vi "Add Abstract Message Attribute.vi"(8 "error in (no error)":errorcluster, 10 "Abstract Message Path":path, 11 "Target Actor in":refnum<vi>) -> (0 "error out":errorcluster, 2 "Abstract Message Control":refnum<vi>)   [LabVIEW 2020, in "Message Maker.lvlib"]
uses:
  Message Maker.lvlib
  <vilib>/Utility/miscctls.llb/LVPointTypeDef.ctl
  <vilib>/Utility/miscctls.llb/LVPositionTypeDef.ctl
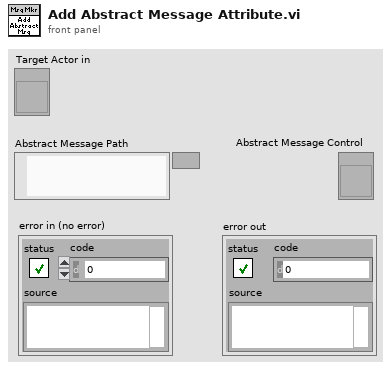
[diagram p1: front panel]
types:
  T1 = typedef "LVPositionTypeDef.ctl" = cluster{"Left":i32, "Top":i32}
  T2 = typedef "LVPointTypeDef.ctl" = cluster{"Horizontal":i16, "Vertical":i16}
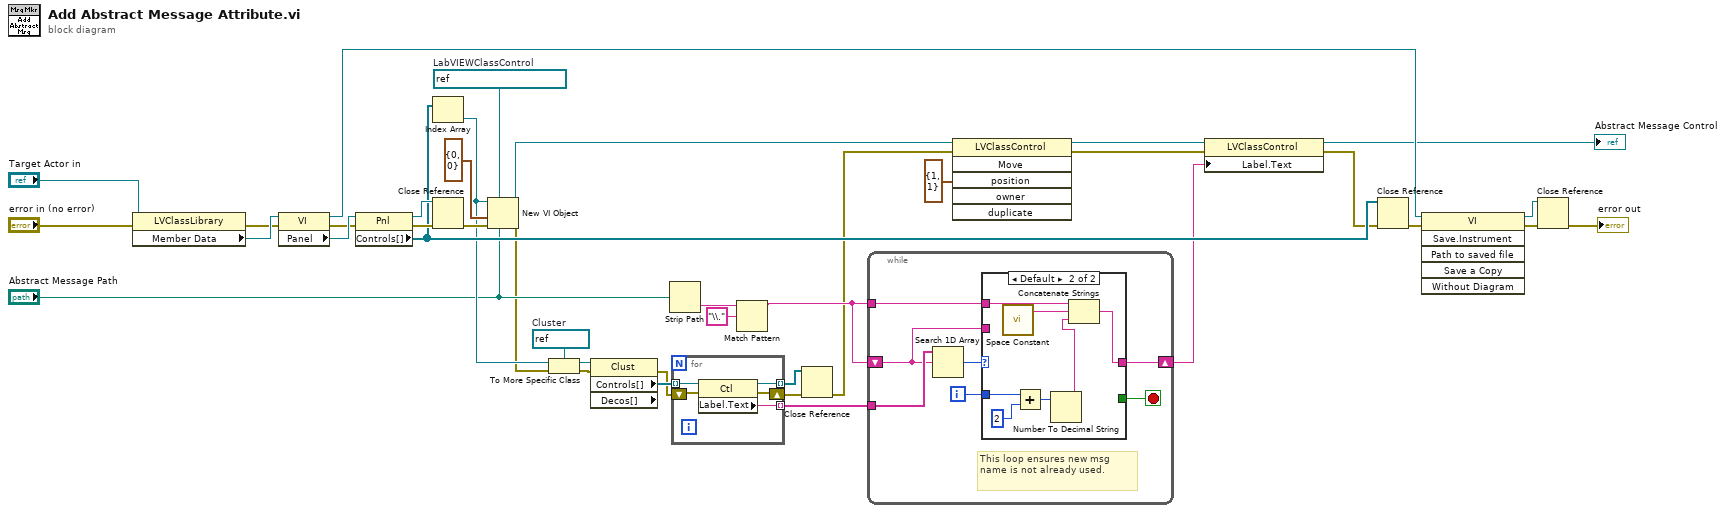
[diagram p0: block diagram]
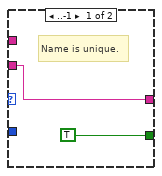
[diagram p2: hidden frame]
diagram:
  w17 = refnum<vi> refnum  # Cluster
  w25 = refnum<vi> refnum  # LabVIEWClassControl
  n1 = property class="LVClassLibrary"(reference="Target Actor in", error in="error in (no error)") -> (error out=w31:errorcluster, "Member Data"=w33:refnum<vi>)  [unwired: 1 out]
  n2 = property class="VI"(reference=w33, error in=w31) -> (reference out=w36:refnum<vi>, error out=w32:errorcluster, "Panel"=w37:refnum<vi>)
  n3 = property class="Pnl"(reference=w37, error in=w32) -> (reference out=w29:refnum<vi>, error out=w30:errorcluster, "Controls[]"=w23:refnum<vi>[])
  n4 = Index Array(array=w23) -> (element=w18:refnum<vi>)  [unwired: 1 in]
  n5 = Close Reference(reference=w29, error in (no error)=w30) -> (error out=w28:errorcluster)
  n6 = New VI Object(vi object class=w25, owner refnum=w18, position/next to=T2 {"Horizontal"=0, "Vertical"=0} ("location"), 6:"Abstract Message Path", 8:w28) -> (object refnum=w3:refnum<vi>, 0:w7:errorcluster)  [unwired: 3 in]
  n7 = To More Specific Class(target class=w17, reference=w18, error in=w7) -> (specific class reference=w6:refnum<vi>, error out=w11:errorcluster)
  n8 = property class="Clust" props=["Controls[]", "Decos[]"](reference=w6, error in=w11) -> (error out=w10:errorcluster, "Controls[]"=w16:refnum<vi>[])  [unwired: 2 out]
  n9 = Strip Path(path="Abstract Message Path") -> (name=w21:string)  [unwired: 1 out]
  n10 = for {
    tunnel: w16 -> [w44] mode=indexing
    tunnel: [w43] -> w15 mode=indexing
    shift-right: [w41] -> w9
    shift-left: w10 -> [w42]
    tunnel: [w40] -> w8 mode=indexing
    n11 = property class="Ctl"(reference=w44, error in=w42) -> (reference out=w40:refnum<vi>, error out=w41:errorcluster, "Label.Text"=w43:string)
  }
  n12 = Match Pattern(string=w21, regular expression="\\.") -> (before substring=w13:string)  [unwired: 1 in, 3 out]
  n13 = Close Reference(reference=w8, error in (no error)=w9) -> (error out=w2:errorcluster)
  n14 = while {
    tunnel: w13 -> [w49]
    shift-right: [w47] -> w12
    shift-left: w13 -> [w45]
    tunnel: w15 -> [w51]
    i -> [w48]
    stop <- w46 stop-if-true
    # "This loop ensures new msg name is not already used."
    n15 = Search 1D Array(1D array=w51, element=w45) -> (index of element=w50:i32)  [unwired: 1 in]
    n16 = case shown="Default" w50 {
      tunnel: w49 -> [_ w60]
      tunnel: w45 -> [w53 _]
      tunnel: w48 -> [_ w58]
      tunnel: [w53 w55] -> w47
      tunnel: [TRUE _] -> w46
      frame ..-1 {
        # "Name is unique."
      }
      frame Default {
        n17 = call <vilib>:"Space Constant.vi"() -> ("String"=w59:string)
        n18 = Add(x=w58, y=2) -> (x+y=w56:i32)
        n19 = Number To Decimal String(number=w56) -> (decimal integer string=w54:string)  [unwired: 1 in]
        n20 = Concatenate Strings(w60, w59, w54) -> (w55:string)
      }
    }
  }
  n21 = invoke class="LVClassControl" method="Move"(reference=w3, error in=w2, "position"=T1 {"Left"=1, "Top"=1}) -> (reference out=w4:refnum<vi>, error out=w1:errorcluster)  [unwired: 3 in, 4 out]
  n22 = property class="LVClassControl"(reference=w4, error in=w1, "Label.Text"=w12) -> (reference out=→"Abstract Message Control":refnum<vi>, error out=w19:errorcluster)
  n23 = Close Reference(reference=w23, error in (no error)=w19) -> (error out=w27:errorcluster)
  n24 = invoke class="VI" method="Save.Instrument"(reference=w36, error in=w27) -> (reference out=w34:refnum<vi>, error out=w35:errorcluster)  [unwired: 4 in, 4 out]
  n25 = Close Reference(reference=w34, error in (no error)=w35) -> (error out=→"error out":errorcluster)
